vi "play-simple-force-mapping.vi"() -> ()   [LabVIEW 2017]
uses:
  <vilib>/userdefined/High Color/nirio_resource_hc.ctl
  <vilib>/FPGAPlugInAG/cRIO-9082/niLvFpga_Open_cRIO-9082.vi
  <vilib>/rvi/interface/common/dynamic/niFpgaDynamicAddResources.vi
  <vilib>/FPGAPlugInAG/Dynamic/niLvFpga_Reset_Dynamic.vi
  <vilib>/rvi/interface/common/niFpgaWaitOnOcc.vi
  <vilib>/Utility/error.llb/Error Cluster From Error Code.vi
  <vilib>/rvi/errors/niLvFpgaAdjustHostInterfaceError.vi
  <vilib>/FPGAPlugInAG/Dynamic/niLvFpga_Run_Dynamic.vi
  <vilib>/Utility/file.llb/Write Delimited Spreadsheet (DBL).vi
  <vilib>/FPGAPlugInAG/Dynamic/niLvFpga_Close_Dynamic.vi
  <vilib>/rvi/interface/nirviOpenFPGA/nirviOpenFPGA.xnode
  FPGA Bitfiles/afmimagingcontro_FPGATargetSPARTA_simple-force-map_FwCwu-swAI0.lvbitx
  <vilib>/rvi/interface/nirviMethod/nirviMethod.xnode
  <vilib>/rvi/interface/nirviReadWriteControl/nirviReadWriteControl.xnode
  <vilib>/rvi/interface/nirviCloseFPGA/nirviCloseFPGA.xnode
  <vilib>/FPGAPlugInAG/Dynamic/niLvFpga_ConfigureFifo_Dynamic.vi
  <vilib>/rvi/errors/niLvFpgaMergeErrorWithErrorCode.vi
  <vilib>/rvi/interface/Simulation/niFpgaSimulationCallBeginRW.vi
  <vilib>/FPGAPlugInAG/Dynamic/niLvFpga_ReadFifo_Dynamic.vi
  NiFpgaLv.dll
  controls/expMetaData.ctl
  <userlib>/_matio/level5.lvlib
  <userlib>/_matio/level5/Public/Write/Append Data Element.llb/Append Data Element (Anything).vi
panel:
  out "Current Case 2":i16
  out "Numeric":i32
  in  "sysID_Z_axis_params":T1={"TOL"=0.3, "ramp-rate"=-5e-05, "z-u-max"=0.0, "offset"=0.0, "Ki"=0.005, "Z-error-threshold"=0.05, "Z-settled-samples\nthreshold "=0, "z_UP"=0.0, "zup-N"=0}
  out "result string":string
  out "boolean  indicators":T2
  in  "Tab Control":enum32{"Main Settings", "Host Debug"}(tab)
  in  "init Z up":sgl step=0.5
  in  "trigger-0":bool
  in  "outputData":path=path "C:/Users/arnold/Documents/labview/afm_imaging/data/data-out.csv"
  in  "TsTicks":u32=1600
  out "e(0) (threshhold init)":fxp<+/-,16,5>
  in  "z-down-max":fxp<+/-,32,16>
  out "Current Case":i16
  out "iter":i32
  out "size(s)":i32
  out "y iter":i32
  out "size(s) 2":i32[](array[numeric])
  out "Array":i32[][](array[numeric])
  out "z-control":dbl[](graph)
  out "z-error":dbl[](graph)
  in  "STOP":bool
  # "- If collect all = fasle and collect move = false,\nwe only collect measurement data.\n- If collect all = false, and collect move = true,\nwe collect measurement and move data.\n- If collect all = true, we collect everything."
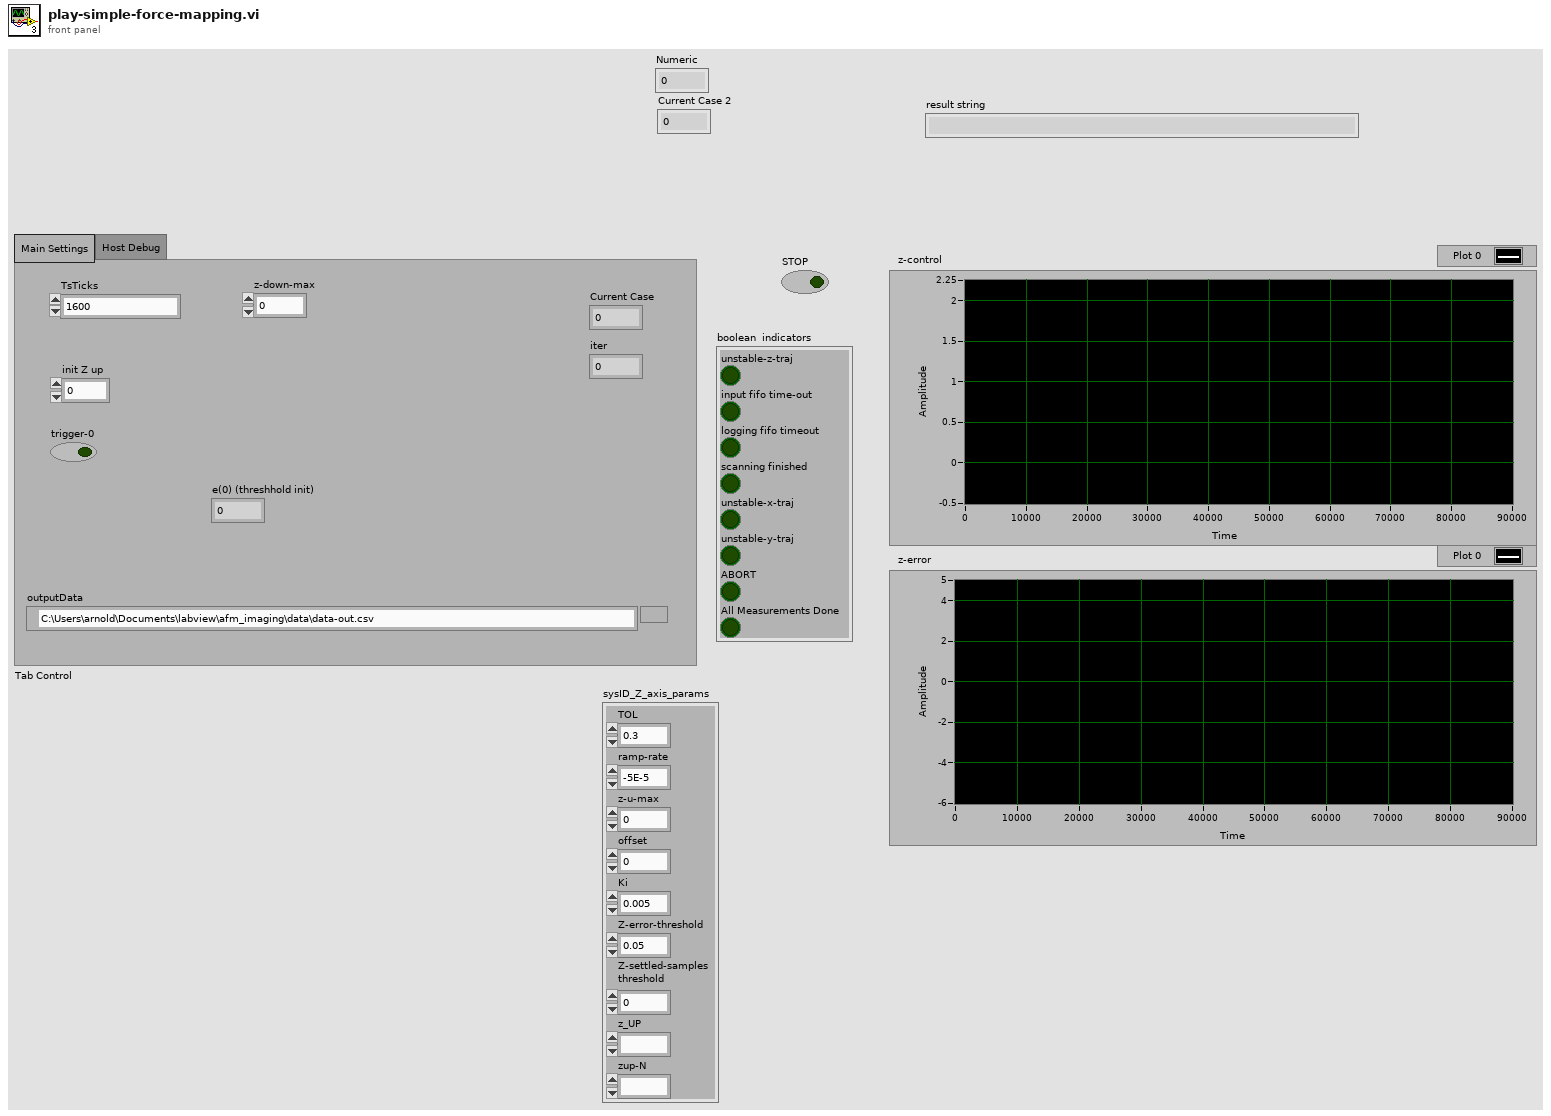
[diagram p1: front panel]
types:
  T1 = cluster{"TOL":sgl, "ramp-rate":sgl, "z-u-max":sgl, "offset":sgl, "Ki":sgl, "Z-error-threshold":sgl, "Z-settled-samples\nthreshold ":i16, "z_UP":fxp<+/-,16,5>, "zup-N":i16}
  T2 = cluster{"unstable-z-traj":bool, "input fifo time-out":bool, "logging fifo timeout":bool, "scanning finished":bool, "unstable-x-traj":bool, "unstable-y-traj":bool, "ABORT":bool, "All Measurements Done":bool}
  T3 = typedef "nirio_resource_hc.ctl" = tag
  T4 = enum16{"open", "replace", "create", "open or create", "replace or create", "replace or create with confirmation"}
  T5 = typedef "expMetaData.ctl" = cluster{"xy_error_threshold":sgl, "xy_settled_samples_threshold":i16, "Ki_xy":sgl, "state_counts":dbl[], "TOL":sgl, "ramp_rate":sgl, "z_u_max":sgl, "setpoint":sgl, "Ki":sgl, "Z_error_threshold":sgl, "Z_settled_samples_threshold ":i16, "z_UP":sgl, "zup_N":i16}
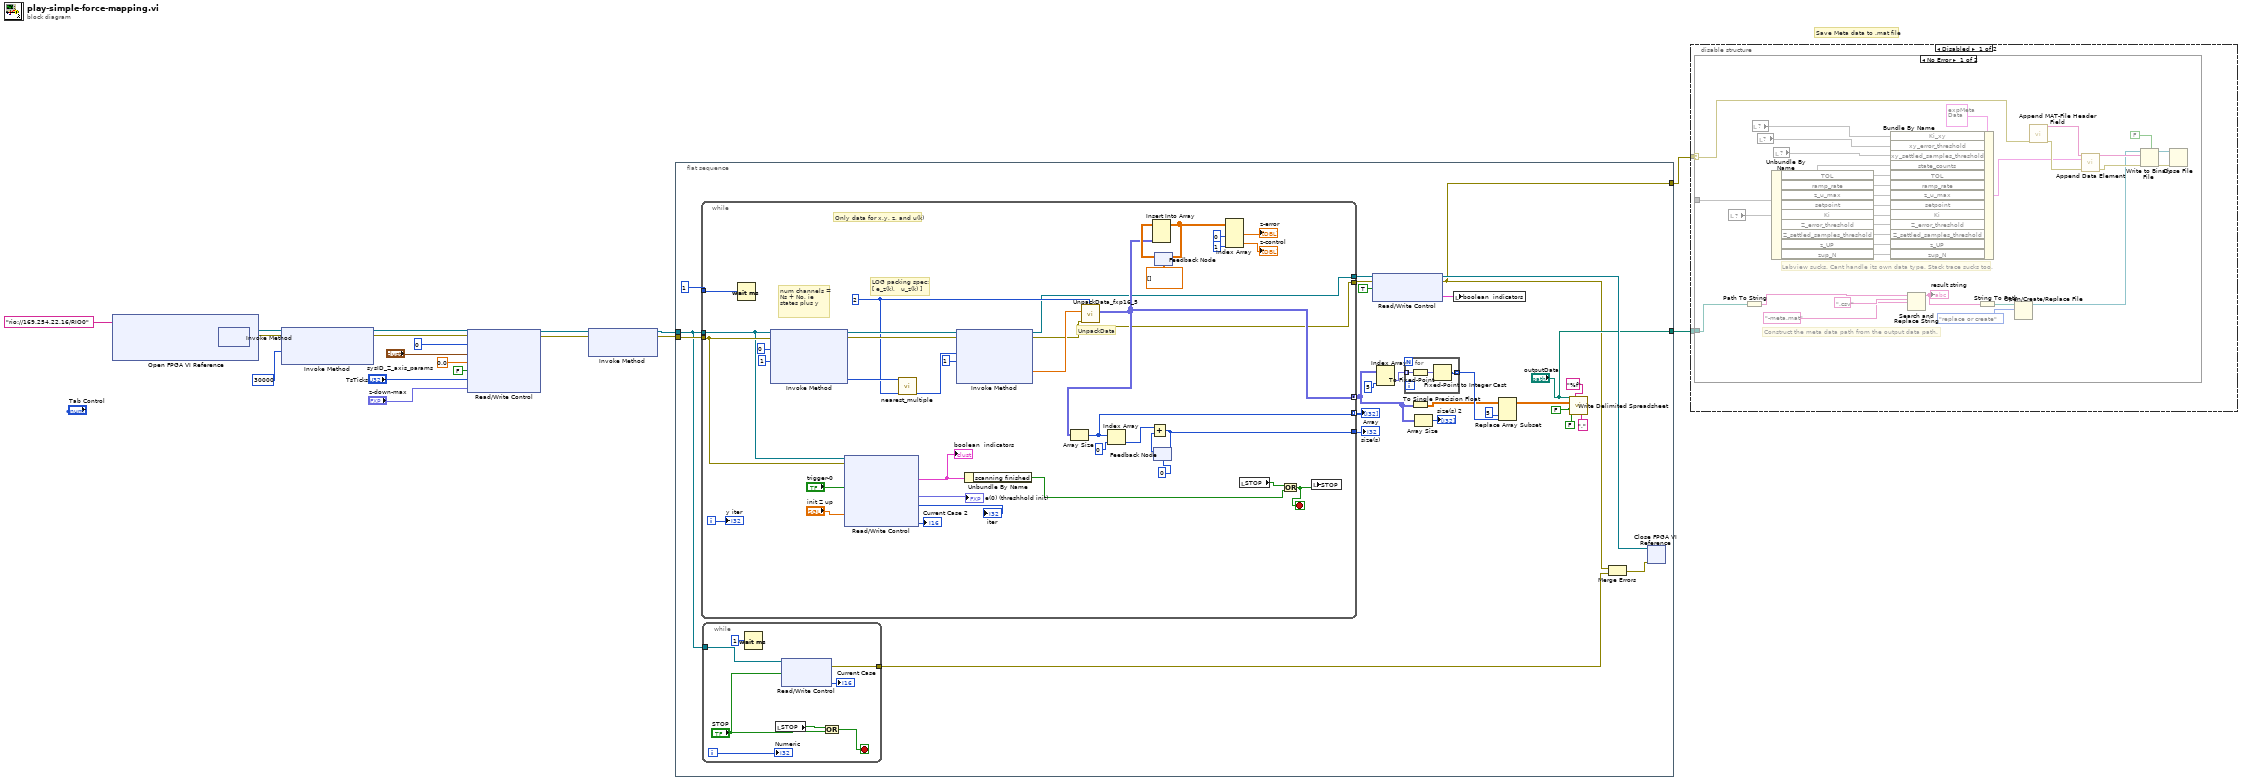
[diagram p0: block diagram]
diagram:
  # "Save Meta data to .mat file"
  n1 = xnode "Open FPGA VI Reference"("resource name"=T3 "rio://169.254.22.16/RIO0") -> ("FPGA VI Reference Out"=w19:refnum<k20>, "error out"=w18:errorcluster)  [unwired: 1 in]
  n2 = xnode "Invoke Method"("FPGA VI Reference In"=w19, "error in"=w18) -> ("FPGA VI Reference Out"=w16:refnum<k20>, "error out"=w15:errorcluster)
  n3 = xnode "Invoke Method"("FPGA VI Reference In"=w16, "error in"=w15, "Requested Depth"=30000) -> ("FPGA VI Reference Out"=w6:refnum<k20>, "error out"=w5:errorcluster)  [unwired: 1 out]
  n4 = xnode "Read/Write Control"("FPGA VI Reference In"=w6, "error in"=w5, "initial case"=i16 0, "sysID_Z_axis_params"="sysID_Z_axis_params", "init Z up"=sgl 0.0 ("u(0)"), "trigger-0"=FALSE, "TsTicks"="TsTicks", "z-down-max"="z-down-max") -> ("FPGA VI Reference Out"=w2:refnum<k20>, "error out"=w1:errorcluster)
  n5 = xnode "Invoke Method"("FPGA VI Reference In"=w2, "error in"=w1) -> ("FPGA VI Reference Out"=w4:refnum<k20>, "error out"=w3:errorcluster)  [unwired: 1 in]
  n6 = flat-sequence {
    tunnel: w3 -> [w44]
    tunnel: w4 -> [w34]
    tunnel: [w21] -> w9
    tunnel: ["outputData"] -> w10
    frame #0 {
      n7 = while {
        tunnel: 1 -> [w95]
        tunnel: w34 -> [w84]
        tunnel: w44 -> [w85]
        tunnel: [w62] -> w39
        tunnel: [w67] -> w26 mode=concatenating
        tunnel: [w82] -> w45
        tunnel: [w65] -> w38
        tunnel: [w74] -> w33 mode=indexing
        i -> [w83]
        stop <- w75 stop-if-true
        w68 = u32 2 ("y")
        # "LOG packing spec:\n[ e_z(k),   u_z(k) ]"
        # "num channels = Ns + No, ie states plus y"
        # "Only data for x,y, z, and u(k)"
        # "UnpackData"
        n8 = Wait (ms)(milliseconds to wait=w95) -> ()  [unwired: 1 out]
        n9 = xnode "Invoke Method"("FPGA VI Reference In"=w84, "error in"=w85, "Number of Elements"=0 ("Timeout (ms)"), "Timeout (ms)"=1) -> ("FPGA VI Reference Out"=w91:refnum<k20>, "error out"=w92:errorcluster, "Elements Remaining"=w79:u32)  [unwired: 1 out]
        n10 = xnode "Read/Write Control"("FPGA VI Reference In"=w84, "error in"=w85, "trigger-0"="trigger-0", "init Z up"="init Z up") -> ("boolean  indicators"=w77:T2, "e(0) (threshhold init)"=→"e(0) (threshhold init)":fxp<+/-,16,5>, "iter"=→"iter":i32, "Current Case"=→"Current Case 2":i16)  [unwired: 1 in, 2 out]
        "boolean  indicators" <- w77
        n11 = call "nearest_multiple.vi"("numChan"=w68, "N"=w79) -> ("(int) y*floor(x/y)"=w78:u64)  [unwired: 9 in]
        n12 = xnode "Invoke Method"("FPGA VI Reference In"=w91, "error in"=w92, "Number of Elements"=w78, "Timeout (ms)"=1) -> ("FPGA VI Reference Out"=w62:refnum<k20>, "error out"=w65:errorcluster, "Data"=w66:sgl[])  [unwired: 1 out]
        n13 = Unbundle By Name(w77) -> ("scanning finished"=w64:bool)
        n14 = call "UnpackData_fxp16_5.vi"("NumChannels"=w68, "error In"=w65, "1D Data In"=w66) -> ("2D Data Out"=w67:fxp<+/-,16,5>[][])  [unwired: 7 in, 1 out]
        n15 = Array Size(array=w67) -> (size(s)=w74:i32[])
        n16 = Index Array(array=w74, index=0) -> (element=w87:i32)
        n17 = feedback #1(0) -> (w88:i32)
        n18 = Add(x=w87, y=w88) -> (x+y=w82:i32)
        n19 = feedback-in #1(w82) -> ()
        n20 = feedback #2(dbl[][] []) -> (w72:dbl[][])
        n21 = Insert Into Array(array=w72, new element=w67) -> (w69:dbl[][])  [unwired: 2 in]
        n22 = feedback-in #2(w69) -> ()
        n23 = Index Array(array=w69, index (col) #1=0 ("disabled index (col)"), index (col) #2=1 ("index (col)")) -> (element #1=→"z-error":dbl[], element #2=→"z-control":dbl[])  [unwired: 2 in]
        n24 = local read "STOP"() -> (w76:bool)
        n25 = Or(x=w76, y=w64) -> (x .or. y?=w75:bool)
        n26 = local write "STOP"(w75) -> ()
        "y iter" <- w83
      }
      "size(s)" <- w45
      "Array" <- w33
      n27 = while {
        tunnel: w34 -> [w57]
        tunnel: [w50] -> w23
        i -> [w51]
        stop <- w53 stop-if-true
        n28 = Wait (ms)(milliseconds to wait=u32 1) -> ()  [unwired: 1 out]
        n29 = local read "STOP"() -> (w54:bool)
        n30 = xnode "Read/Write Control"("FPGA VI Reference In"=w57, "ABORT"="STOP") -> ("error out"=w50:errorcluster, "Current Case"=→"Current Case":i16)  [unwired: 1 in, 1 out]
        n31 = Or(x=w54, y="STOP") -> (x .or. y?=w53:bool)
        "Numeric" <- w51
      }
      n32 = xnode "Read/Write Control"("FPGA VI Reference In"=w39, "error in"=w38, "ABORT"=TRUE) -> ("FPGA VI Reference Out"=w36:refnum<k20>, "error out"=w21:errorcluster, "boolean  indicators"=w32:T2)
      n33 = Index Array(array=w26, index (col)=5) -> (element=w30:fxp<+/-,16,5>[])  [unwired: 1 in]
      n34 = for {
        tunnel: w30 -> [w48] mode=indexing
        tunnel: [w49] -> w28 mode=indexing
        n35 = To Fixed-Point(number=w48) -> (fixed-point=w47:fxp<+/-,16,5>)  [unwired: 1 in]
        n36 = Fixed-Point to Integer Cast(1:w47) -> (0:w49:i16)
      }
      n37 = To Single Precision Float(number=w26) -> (single precision float=w25:sgl[][])
      n38 = Array Size(array=w26) -> (size(s)=→"size(s) 2":i32[])
      n39 = local write "boolean  indicators"(w32) -> ()
      n40 = Replace Array Subset(array=w25, new element=w28, index (col)=5) -> (w27:sgl[][])  [unwired: 1 in]
      n41 = call-poly <vilib>:"Write Delimited Spreadsheet.vi"("file path (dialog if empty)"="outputData", "format (%.3f)"="%f", "2D data"=w27, "append to file? (new file:F)"=FALSE, "transpose? (no:F)"=FALSE, "delimiter (\\t)"=",") -> ()  [unwired: 8 in, 2 out]
      n42 = Merge Errors(w21, w23) -> (w22:errorcluster)
      n43 = xnode "Close FPGA VI Reference"("FPGA VI Reference In"=w36, "error in"=w22) -> ()  [unwired: 1 out]
    }
  }
  n44 = disable-structure shown="Disabled" {
    disable-tunnel: w10 -> [w97 _]
    disable-tunnel: w9 -> [w96 _]
    frame Disabled {
      n45 = case shown="No Error" w96 {
        selector: w96 -> [w118 _]
        tunnel: w97 -> [w99 _]
        tunnel: _ -> [w104 _]
        frame No Error {
          # "Construct the meta data path from the output data path."
          # "Labview sucks. Cant handle its own data type. Stack trace sucks too."
          n46 = local read item#-1() -> (w103)
          n47 = Path To String(path=w99) -> (string=w121:string)
          n48 = local read item#-1() -> (w102)
          n49 = local read item#-1() -> (w101)
          n50 = Unbundle By Name(w103) -> ("TOL"=w114, "ramp_rate"=w113, "z_u_max"=w112, "setpoint"=w111, "Ki"=w110, "Z_error_threshold"=w109, "Z_settled_samples_threshold"=w108, "z_UP"=w107, "zup_N"=w106)
          n51 = local read item#-1() -> (w100)
          n52 = Bundle By Name(cluster=T5 {"xy_error_threshold"=0.1, "xy_settled_samples_threshold"=200, "Ki_xy"=0.005, "state_counts"=[], "TOL"=0.3, "ramp_rate"=-5e-06, "z_u_max"=5.0, "setpoint"=0.0, "Ki"=0.001, "Z_error_threshold"=0.0, "Z_settled_samples_threshold "=0, "z_UP"=1.5, "zup_N"=5000} ("ExpMetaData"), "Ki_xy"=w102, "xy_error_threshold"=w101, "xy_settled_samples_threshold"=w100, "state_counts"=w104, "TOL"=w114, "ramp_rate"=w113, "z_u_max"=w112, "setpoint"=w111, "Ki"=w110, "Z_error_threshold"=w109, "Z_settled_samples_threshold"=w108, "z_UP"=w107, "zup_N"=w106) -> (w115:T5)
          n53 = Search and Replace String(input string=w121, search string=".csv", replace string="-meta.mat" ("replace string (\"\")")) -> (result string=w120:string)  [unwired: 5 in, 3 out]
          "result string" <- w120
          n54 = String To Path(string=w120) -> (path=w117:path)
          n55 = Open/Create/Replace File(file path (use dialog)=w117, operation (0:open)=T4."replace or create") -> (refnum out=w116:refnum<file>)  [unwired: 4 in, 2 out]
          n56 = call <userlib>:"Append MAT-File Header Field.vi"("error"=w118) -> ("result string"=w129:string, "error out"=w119:errorcluster)  [unwired: 13 in]
          n57 = call-poly <userlib>:"Append Data Element.vi"("initial string"=w129, "data"=w115, "error in (no error)"=w119) -> ("result string"=w127:string, "error out"=w128:errorcluster)  [unwired: 11 in]
          n58 = Write to Binary File(file (use dialog)=w116, data=w127, error in=w128, 5:FALSE ("prepend array or string size? (T)")) -> (refnum out=w124:refnum<file>, error out=w125:errorcluster)  [unwired: 2 in, 1 out]
          n59 = Close File(refnum=w124, error in=w125) -> ()  [unwired: 2 out]
        }
        frame Error {
        }
      }
    }
    frame Enabled {
    }
  }
